vi "Release Tree Data Priv.vi"(0 "Data":variant) -> ()   [LabVIEW 2016, in "Tree Manager.lvclass"]
uses:
  Tree Manager.lvclass
  Tree Data/Tree Data.lvclass
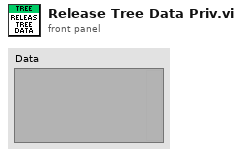
[diagram p1: front panel]
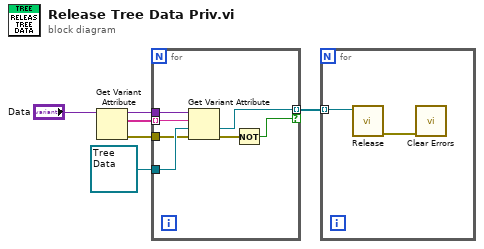
[diagram p0: block diagram]
diagram:
  n1 = Get Variant Attribute(Variant="Data") -> (duplicate Variant=w2:variant, names=w3:string[], error out=w1:errorcluster)  [unwired: 3 in, 1 out]
  n2 = for {
    tunnel: w2 -> [w13]
    tunnel: w3 -> [w12] mode=indexing
    tunnel: refnum<class "Tree Data.lvclass"> refnum ("Tree Data.lvclass") -> [w11]
    tunnel: [w9] -> w5 mode=indexing if=w8
    tunnel: w1 -> [w7]
    n3 = Get Variant Attribute(Variant=w13, name=w12, default value (empty Variant)=w11, error in=w7) -> (value=w9:refnum<class "Tree Data.lvclass">, error out=w10:errorcluster)  [unwired: 2 out]
    n4 = Not(x=w10) -> (.not. x?=w8:bool)
  }
  n5 = for {
    tunnel: w5 -> [w15] mode=indexing
    n6 = call-dynamic "Release.vi"("Tree Data In"=w15) -> ("Error Out"=w14:errorcluster)  [unwired: 10 in]
    n7 = call <vilib>:"Clear Errors.vi"("error in (no error)"=w14) -> ()  [unwired: 5 in, 2 out]
  }
